vi "PhotonPoseEstimator_Execute.vi"(7 "Configuration":T12={"Primary Strategy"=enum."LOWEST_AMBIGUITY", "Camera"="", "Initial Pose"={"Translation3d"={"X"=0.0, "Y"=0.0, "Z"=0.0}, "Rotation3d"={"Q_quaternion"={"R"=1.0, "V"=[0.0, 0.0, 0.0]}}}, "HighestAmbiguity"=0.0, "RobotToCamera"={"TRANSLATION3D"={"X"=0.0, "Y"=0.0, "Z"=0.0}, "ROTATION3D"={"Q_quaternion"={"R"=1.0, "V"=[0.0, 0.0, 0.0]}}, "XF"=FALSE}, "FallBack Strategy"=enum."LOWEST_AMBIGUITY", "BaseNTName"="/photonvision"} {"RobotToCamera"."TRANSLATION3D"."Z" format="%14.3f"; "RobotToCamera"."TRANSLATION3D"."Y" format="%14.3f"; "RobotToCamera"."TRANSLATION3D"."X" format="%14.3f"; "Initial Pose"."Translation3d"."Z" format="%14.3f"; "Initial Pose"."Translation3d"."Y" format="%14.3f"; "Initial Pose"."Translation3d"."X" format="%14.3f"}, 8 "AprilTagFieldLayout":T1={"AprilTagMap"={}, "FieldLength"=0.0, "FieldWidth"=0.0, "OriginPosition "=enum."kBlueAllianceWallRightSide,", "OriginPose3d"={"Translation3d"={"X"=0.0, "Y"=0.0, "Z"=0.0}, "Rotation3d"={"Q_quaternion"={"R"=1.0, "V"=[0.0, 0.0, 0.0]}}}} {"OriginPose3d"."Translation3d"."Z" format="%14.3f"; "OriginPose3d"."Translation3d"."Y" format="%14.3f"; "OriginPose3d"."Translation3d"."X" format="%14.3f"}, 9 "ReferencePose":T3={"Translation3d"={"X"=0.0, "Y"=0.0, "Z"=0.0}, "Rotation3d"={"Q_quaternion"={"R"=1.0, "V"=[0.0, 0.0, 0.0]}}} {"Translation3d"."Z" format="%14.3f"; "Translation3d"."Y" format="%14.3f"; "Translation3d"."X" format="%14.3f"}, 10 "PIpeline Has \nNew Results":bool, 11 "PipelineResult":T14={"Targets"=[], "PhotonMultiTargetPNPResult"={"PhotonPNPResult"={"IsPresent"=FALSE, "bestReprojErr"=0.0, "altReprojErr"=0.0, "ambiguity"=0.0, "Best"={"TRANSLATION3D"={"X"=0.0, "Y"=0.0, "Z"=0.0}, "ROTATION3D"={"Q_quaternion"={"R"=1.0, "V"=[0.0, 0.0, 0.0]}}, "XF"=FALSE}, "Alt"={"TRANSLATION3D"={"X"=0.0, "Y"=0.0, "Z"=0.0}, "ROTATION3D"={"Q_quaternion"={"R"=1.0, "V"=[0.0, 0.0, 0.0]}}, "XF"=FALSE}}, "FiducialIDsUsed"=[]}, "PhotonPipelineMetadata"={"CaptureTimestampMicros"=0, "PublishTimestampMicros"=0, "SequenceID"=0, "TimeSinceLastPong"=0}} {"PhotonMultiTargetPNPResult"."PhotonPNPResult"."Alt"."TRANSLATION3D"."Z" format="%14.3f"; "PhotonMultiTargetPNPResult"."PhotonPNPResult"."Alt"."TRANSLATION3D"."Y" format="%14.3f"; "PhotonMultiTargetPNPResult"."PhotonPNPResult"."Alt"."TRANSLATION3D"."X" format="%14.3f"; "PhotonMultiTargetPNPResult"."PhotonPNPResult"."Best"."TRANSLATION3D"."Z" format="%14.3f"; "PhotonMultiTargetPNPResult"."PhotonPNPResult"."Best"."TRANSLATION3D"."Y" format="%14.3f"; "PhotonMultiTargetPNPResult"."PhotonPNPResult"."Best"."TRANSLATION3D"."X" format="%14.3f"; "Targets"."AltCameraToTarget"."TRANSLATION3D"."Z" format="%14.3f"; "Targets"."AltCameraToTarget"."TRANSLATION3D"."Y" format="%14.3f"; "Targets"."AltCameraToTarget"."TRANSLATION3D"."X" format="%14.3f"; "Targets"."BestCameraToTarget"."TRANSLATION3D"."Z" format="%14.3f"; "Targets"."BestCameraToTarget"."TRANSLATION3D"."Y" format="%14.3f"; "Targets"."BestCameraToTarget"."TRANSLATION3D"."X" format="%14.3f"}) -> (0 "TimeStamp_Seconds":dbl, 1 "New Pose Found":bool, 2 "EstimatedPose2d":T8={"TRANSLATION"={"X"=0.0, "Y"=0.0}, "ROTATION"={"VALUE"=0.0, "COS"=1.0, "SIN"=0.0}} {"ROTATION"."SIN" format="%13.4f"; "ROTATION"."COS" format="%13.4f"; "ROTATION"."VALUE" format="%13.4f"; "TRANSLATION"."Y" format="%14.3f"; "TRANSLATION"."X" format="%14.3f"}, 3 "EstimatedPose3d":T3={"Translation3d"={"X"=0.0, "Y"=0.0, "Z"=0.0}, "Rotation3d"={"Q_quaternion"={"R"=1.0, "V"=[0.0, 0.0, 0.0]}}} {"Translation3d"."Z" format="%14.3f"; "Translation3d"."Y" format="%14.3f"; "Translation3d"."X" format="%14.3f"}, 4 "Strategy Used":T11, 5 "PhotonEstimatedRobotPose":T20={"EstimatedPose"={"Translation3d"={"X"=0.0, "Y"=0.0, "Z"=0.0}, "Rotation3d"={"Q_quaternion"={"R"=1.0, "V"=[0.0, 0.0, 0.0]}}}, "TimeStamp_Seconds"=0.0, "targetsUsed"=[], "Strategy"=enum."LOWEST_AMBIGUITY"} {"targetsUsed"."AltCameraToTarget"."TRANSLATION3D"."Z" format="%14.3f"; "targetsUsed"."AltCameraToTarget"."TRANSLATION3D"."Y" format="%14.3f"; "targetsUsed"."AltCameraToTarget"."TRANSLATION3D"."X" format="%14.3f"; "targetsUsed"."BestCameraToTarget"."TRANSLATION3D"."Z" format="%14.3f"; "targetsUsed"."BestCameraToTarget"."TRANSLATION3D"."Y" format="%14.3f"; "targetsUsed"."BestCameraToTarget"."TRANSLATION3D"."X" format="%14.3f"; "EstimatedPose"."Translation3d"."Z" format="%14.3f"; "EstimatedPose"."Translation3d"."Y" format="%14.3f"; "EstimatedPose"."Translation3d"."X" format="%14.3f"}, 6 "out PhotonPoseEstimator":T21={"LastPose"={"Translation3d"={"X"=0.0, "Y"=0.0, "Z"=0.0}, "Rotation3d"={"Q_quaternion"={"R"=1.0, "V"=[0.0, 0.0, 0.0]}}}, "ReferencePose"={"Translation3d"={"X"=0.0, "Y"=0.0, "Z"=0.0}, "Rotation3d"={"Q_quaternion"={"R"=1.0, "V"=[0.0, 0.0, 0.0]}}}, "FieldTags"={"AprilTagMap"={}, "FieldLength"=0.0, "FieldWidth"=0.0, "OriginPosition "=enum."kBlueAllianceWallRightSide,", "OriginPose3d"={"Translation3d"={"X"=0.0, "Y"=0.0, "Z"=0.0}, "Rotation3d"={"Q_quaternion"={"R"=1.0, "V"=[0.0, 0.0, 0.0]}}}}, "PrimaryStratety"=enum."LOWEST_AMBIGUITY", "Camera"="", "RobotToCamera"={"TRANSLATION3D"={"X"=0.0, "Y"=0.0, "Z"=0.0}, "ROTATION3D"={"Q_quaternion"={"R"=1.0, "V"=[0.0, 0.0, 0.0]}}, "XF"=FALSE}, "ReportedErrors"=[], "HighestAmbiguity"=10.0, "MultiTagFallbackStrategy"=enum."LOWEST_AMBIGUITY", "PoseCacheTimeoutSec"=-1.0, "PhotonTargetModel"={"Vertices"=[], "IsPlaner"=FALSE, "IsSpherical"=FALSE}, "BaseNTName"="/photonvision", "HeadingBuffer"={"TimeStamps"=[], "RotationValues"=[], "Min_TimeStamp"=0.0, "Max_TimeStamp"=0.0, "ItemCount"=0, "MaxBufferTime"=0.0}} {"HeadingBuffer"."RotationValues"."SIN" format="%13.4f"; "HeadingBuffer"."RotationValues"."COS" format="%13.4f"; "HeadingBuffer"."RotationValues"."VALUE" format="%13.4f"; "PhotonTargetModel"."Vertices"."Z" format="%14.3f"; "PhotonTargetModel"."Vertices"."Y" format="%14.3f"; "PhotonTargetModel"."Vertices"."X" format="%14.3f"; "RobotToCamera"."TRANSLATION3D"."Z" format="%14.3f"; "RobotToCamera"."TRANSLATION3D"."Y" format="%14.3f"; "RobotToCamera"."TRANSLATION3D"."X" format="%14.3f"; "FieldTags"."OriginPose3d"."Translation3d"."Z" format="%14.3f"; "FieldTags"."OriginPose3d"."Translation3d"."Y" format="%14.3f"; "FieldTags"."OriginPose3d"."Translation3d"."X" format="%14.3f"; "ReferencePose"."Translation3d"."Z" format="%14.3f"; "ReferencePose"."Translation3d"."Y" format="%14.3f"; "ReferencePose"."Translation3d"."X" format="%14.3f"; "LastPose"."Translation3d"."Z" format="%14.3f"; "LastPose"."Translation3d"."Y" format="%14.3f"; "LastPose"."Translation3d"."X" format="%14.3f"})   [LabVIEW 2019, in "PhotonVisionLib.lvlib"]
doc: "Provided data from polling a camera, update the estimated position of the robot. Returns empty if there are no cameras set or no targets were found from the cameras. \n\nInputs:\n -- PhotonPoseEstimator -- data cluster -- Data guiding how the position determination is done.\n -- PipelineResults -- data cluster -- Data provided from PhotonCamera_GetLatestResults.\n -- HasResults -- boolean - TRUE if targets have been identified in the Pipeline results. This can be provided by PhotonCamera_GetLatestResults.\n -- AprilTagFieldLayout -- data cluster -- Field layout defining the location of April Tags\n\nOutputs:\n - EstimatedPose3d - Pose3d - Estimated 3d position. Only value if NewPoseFound = TRUE\n - EstimatedPose2d - Pose2d - Estimated 2d position. Only value if NewPoseFound = TRUE\n - NewPoseFound -- boolean -- A new position has been determined.\n - TimeStampe - double - Target timestamp (seconds)\n - StrategyUsed -- enum -- The strategy used to determine the pose.\n - PhotonEstimatedRobotPose -- data cluster -- Complete estimated robot position and timestamp data cluster\n -- PhotonPoseEstimator -- data cluster -- Updated data cluster."
uses:
  PhotonVisionLib.lvlib
  TypeDef/PhotonPoseEstimatorType.ctl
  <vilib>/Rock Robotics/WPI/ThirdParty/JAS_Junk/TrajLib/TypeDef/POSE3D.ctl
  <vilib>/Rock Robotics/WPI/ThirdParty/JAS_Junk/TrajLib/TypeDef/TRANSLATION3D.ctl
  <vilib>/Rock Robotics/WPI/ThirdParty/JAS_Junk/TrajLib/TypeDef/ROTATION3D.ctl
  <vilib>/Rock Robotics/WPI/ThirdParty/JAS_Junk/TrajLib/TypeDef/QUATERNION.ctl
  <vilib>/Rock Robotics/WPI/ThirdParty/JAS_Junk/TrajLib/TypeDef/AprilTagFieldLayout.ctl
  <vilib>/Rock Robotics/WPI/ThirdParty/JAS_Junk/TrajLib/TypeDef/AprilTag.ctl
  <vilib>/Rock Robotics/WPI/ThirdParty/JAS_Junk/TrajLib/Enum/AprilTagFieldLayoutOrignPosition_ENUM.ctl
  Enum/PhotonPoseStrategy_ENUM.ctl
  <vilib>/Rock Robotics/WPI/ThirdParty/JAS_Junk/TrajLib/TypeDef/TRANSFORM3D.ctl
  TypeDef/PhotonTargetModel.ctl
  <vilib>/Rock Robotics/WPI/ThirdParty/JAS_Junk/TrajLib/TypeDef/TIME_INTERPOLATABLE_ROTATION2D.ctl
  <vilib>/Rock Robotics/WPI/ThirdParty/JAS_Junk/TrajLib/TypeDef/ROTATION2D.ctl
  TypeDef/PhotonEstimatedRobotPoseType.ctl
  TypeDef/PhotonTrackedTargetType.ctl
  TypeDef/TargetCornerType.ctl
  TypeDef/PhotonPipelineResultType.ctl
  TypeDef/PhotonMultiTargetPNPResultType.ctl
  TypeDef/PhotonPNPResultType.ctl
  TypeDef/PhotonPipelineMetadataType.ctl
  TypeDef/PhotonPoseEstimator_Configuration.ctl
  <vilib>/Rock Robotics/WPI/ThirdParty/JAS_Junk/TrajLib/TypeDef/POSE2D.ctl
  <vilib>/Rock Robotics/WPI/ThirdParty/JAS_Junk/TrajLib/TypeDef/TRANSLATION2D.ctl
  <vilib>/Rock Robotics/WPI/ThirdParty/JAS_Junk/TrajLib/VI/Transform3d_GetTranslation3d.vi
  <vilib>/Rock Robotics/WPI/ThirdParty/JAS_Junk/TrajLib/VI/Transform3d_GetRotation3d.vi
  <vilib>/Rock Robotics/WPI/ThirdParty/JAS_Junk/TrajLib/VI/Rotation3d_Equals.vi
  <vilib>/Rock Robotics/WPI/ThirdParty/JAS_Junk/TrajLib/VI/Translation3d_Equals.vi
  PhotonTargetModel_New_AprilTag36H11.vi
  <vilib>/Rock Robotics/WPI/ThirdParty/JAS_Junk/TrajLib/VI/TimeInterpRotation2d_New.vi
  PhotonPoseEstimator_Update_All.vi
  <vilib>/Rock Robotics/WPI/ThirdParty/JAS_Junk/TrajLib/VI/Pose3d_getTranslation3d.vi
  <vilib>/Rock Robotics/WPI/ThirdParty/JAS_Junk/TrajLib/VI/Pose3d_getRotation3d.vi
  <vilib>/Rock Robotics/WPI/ThirdParty/JAS_Junk/TrajLib/VI/Translation3d_ToTranslation2d.vi
  <vilib>/Rock Robotics/WPI/ThirdParty/JAS_Junk/TrajLib/VI/Rotation3d_ToRotation2d.vi
  <vilib>/Rock Robotics/WPI/ThirdParty/JAS_Junk/TrajLib/Pose2d_New_TRRO.vi
  <vilib>/Rock Robotics/WPI/ThirdParty/JAS_Junk/TrajLib/VI/Rotation3d_GetQuaterion.vi
  <vilib>/Rock Robotics/WPI/ThirdParty/JAS_Junk/TrajLib/VI/Quaternion_Equals.vi
  PhotonTargetModel_New_RectPlanar.vi
  <vilib>/Rock Robotics/WPI/ThirdParty/JAS_Junk/TrajLib/Conv_Inches_Meters.vi
  PhotonPoseEstimator_GetEmptyPose.vi
  PhotonPoseEstimator_Strategy_lowestAmbiguity.vi
  PhotonPoseEstimator_Strategy_closestToCameraHeight.vi
  PhotonPoseEstimator_Strategy_closestToReferencePose.vi
  PhotonPoseEstimator_GetReferencePose.vi
  PhotonPoseEstimator_GetLastPose.vi
  PhotonPoseEstimator_Strategy_averageBestTargets.vi
  PhotonPoseEstimator_Strategy_multiTagOnCoproc.vi
  PhotonPoseEstimator_Strategy_pnpDistanceTrigSolve.vi
  PhotonPoseEstimator_Strategy_constrainedPnpStrategy.vi
  PhotonPipelineResult_GetTimeStampSecs.vi
  <vilib>/Rock Robotics/WPI/ThirdParty/JAS_Junk/TrajLib/Translation2d_Create.vi
  <vilib>/Rock Robotics/WPI/ThirdParty/JAS_Junk/TrajLib/Rotation2d_CreateAngle.vi
  <vilib>/Rock Robotics/WPI/ThirdParty/JAS_Junk/TrajLib/VI/Rotation3d_GetXYZ.vi
  <vilib>/Rock Robotics/WPI/ThirdParty/JAS_Junk/TrajLib/VI/Quaternion_Get_Vect.vi
  <vilib>/Rock Robotics/WPI/ThirdParty/JAS_Junk/TrajLib/VI/Quaternion_Get_W.vi
  <vilib>/Rock Robotics/WPI/ThirdParty/JAS_Junk/TrajLib/VI/Translation3d_Create.vi
  PhotonTargetModel_New.vi
  <vilib>/Rock Robotics/WPI/ThirdParty/JAS_Junk/TrajLib/VI/Rotation3d_Create_AxisAngle.vi
  <vilib>/Rock Robotics/WPI/ThirdParty/JAS_Junk/TrajLib/VI/Pose3d_New.vi
  PhotonPipelineResult_HasTargets.vi
  PhotonPipelineResult_GetTargets.vi
  PhotonTrackedTarget_GetPoseAmbiguity.vi
  PhotonTrackedTarget_GetFiducialId.vi
  PhotonPoseEstimator_GetFieldTags.vi
  <vilib>/Rock Robotics/WPI/ThirdParty/JAS_Junk/TrajLib/VI/AprilTagFieldLayout_GetTagPose.vi
  <vilib>/Rock Robotics/WPI/ThirdParty/JAS_Junk/TrajLib/VI/Pose3d_TransformBy.vi
  PhotonTrackedTarget_GetBestCameraToTarget.vi
  <vilib>/Rock Robotics/WPI/ThirdParty/JAS_Junk/TrajLib/VI/Transform3d_Inverse.vi
  PhotonPoseEstimator_GetRobotToCameraTransform.vi
  PhotonPoseEstimator_GetHighestAmbiguity.vi
  PhotonEstimatedRobotPose_New.vi
  PhotonPoseEstimator_Strategy_closestToCameraHeight_calc.vi
  PhotonTrackedTarget_GetAltCameraToTarget.vi
  PhotonPoseEstimator_Strategy_closestToReferencePose_calc.vi
  PhotonPoseEstimator_Strategy_averageBestTargets_calc.vi
  <vilib>/Rock Robotics/WPI/ThirdParty/JAS_Junk/TrajLib/VI/Rotation3d_Plus.vi
  <vilib>/Rock Robotics/WPI/ThirdParty/JAS_Junk/TrajLib/VI/Translation3d_Plus.vi
  <vilib>/Rock Robotics/WPI/ThirdParty/JAS_Junk/TrajLib/VI/Translation3d_Times.vi
  <vilib>/Rock Robotics/WPI/ThirdParty/JAS_Junk/TrajLib/VI/Rotation3d_Times.vi
  <vilib>/Rock Robotics/WPI/ThirdParty/JAS_Junk/TrajLib/VI/Rotation3d_Create_Default.vi
  <vilib>/Rock Robotics/WPI/ThirdParty/JAS_Junk/TrajLib/VI/Translation3d_Create_Default.vi
  <vilib>/Rock Robotics/WPI/ThirdParty/JAS_Junk/TrajLib/VI/Pose3d_New_Trans3dRot3d.vi
  <vilib>/Rock Robotics/WPI/ThirdParty/JAS_Junk/TrajLib/VI/Pose3d_New_Default.vi
  <vilib>/Rock Robotics/WPI/ThirdParty/JAS_Junk/TrajLib/VI/Pose3d_Plus.vi
  <vilib>/Rock Robotics/WPI/ThirdParty/JAS_Junk/TrajLib/VI/Pose3d_RelativeTo.vi
  <vilib>/Rock Robotics/WPI/ThirdParty/JAS_Junk/TrajLib/VI/AprilTagFieldLayout_GetOriginPosition.vi
  PhotonPipelineResult_GetMultiTagResult.vi
  <vilib>/Rock Robotics/WPI/ThirdParty/JAS_Junk/TrajLib/VI/Quaternion_Get_All.vi
  <vilib>/Rock Robotics/WPI/ThirdParty/JAS_Junk/TrajLib/VI/Quaternion_New.vi
  <vilib>/Rock Robotics/WPI/ThirdParty/JAS_Junk/TrajLib/VI/Vector_Norm.vi
  <vilib>/Rock Robotics/WPI/ThirdParty/JAS_Junk/TrajLib/VecBuilder_ArrayBy1Fill.vi
  <vilib>/Rock Robotics/WPI/ThirdParty/JAS_Junk/TrajLib/VI/AprilTag_GetAll.vi
  <vilib>/Rock Robotics/WPI/ThirdParty/JAS_Junk/TrajLib/VI/Translation3d_RotateBy.vi
  <vilib>/Rock Robotics/WPI/ThirdParty/JAS_Junk/TrajLib/Transform2d_Create_TransRot.vi
  <vilib>/Rock Robotics/WPI/ThirdParty/JAS_Junk/TrajLib/VI/Transform3d_Create_Trans3dRot3d.vi
  <vilib>/Rock Robotics/WPI/ThirdParty/JAS_Junk/TrajLib/VI/Rotation3d_UnaryMinus.vi
  <vilib>/Rock Robotics/WPI/ThirdParty/JAS_Junk/TrajLib/VI/Translation3d_UnaryMinus.vi
  <vilib>/Rock Robotics/WPI/ThirdParty/JAS_Junk/TrajLib/VI/Transform3d_GetXYZ.vi
  <vilib>/Rock Robotics/WPI/ThirdParty/JAS_Junk/TrajLib/VI/Pose3d_getXYZ.vi
  PhotonPoseEstimator_CalcDifference.vi
  <vilib>/Rock Robotics/WPI/ThirdParty/JAS_Junk/TrajLib/VI/Rotation3d_RotateBy.vi
  <vilib>/Rock Robotics/WPI/ThirdParty/JAS_Junk/TrajLib/VI/Translation3d_GetXYZ.vi
  <vilib>/Rock Robotics/WPI/ThirdParty/JAS_Junk/TrajLib/VI/Quaternion_New_Default.vi
  <vilib>/Rock Robotics/WPI/ThirdParty/JAS_Junk/TrajLib/VI/Transform3d_Create_Pose3dPose3d.vi
  <vilib>/Rock Robotics/WPI/ThirdParty/JAS_Junk/TrajLib/MatBuilder_Create.vi
  <vilib>/Rock Robotics/WPI/ThirdParty/JAS_Junk/TrajLib/VI/Quaternion_Times.vi
  <vilib>/Rock Robotics/WPI/ThirdParty/JAS_Junk/TrajLib/VI/Quaternion_Inverse.vi
  <vilib>/Rock Robotics/WPI/ThirdParty/JAS_Junk/TrajLib/VI/Rotation3d_Create_Quaternion.vi
  <vilib>/Rock Robotics/WPI/ThirdParty/JAS_Junk/TrajLib/VI/Translation3d_GetDistance.vi
  <vilib>/Rock Robotics/WPI/ThirdParty/JAS_Junk/TrajLib/VI/Translation3d_Minus.vi
  <vilib>/Rock Robotics/WPI/ThirdParty/JAS_Junk/TrajLib/VI/Rotation3d_Minus.vi
  <vilib>/Rock Robotics/WPI/ThirdParty/JAS_Junk/TrajLib/VI/Quaternion_Normalize.vi
  <vilib>/Rock Robotics/WPI/ThirdParty/JAS_Junk/TrajLib/Trajectory_Library.lvlib
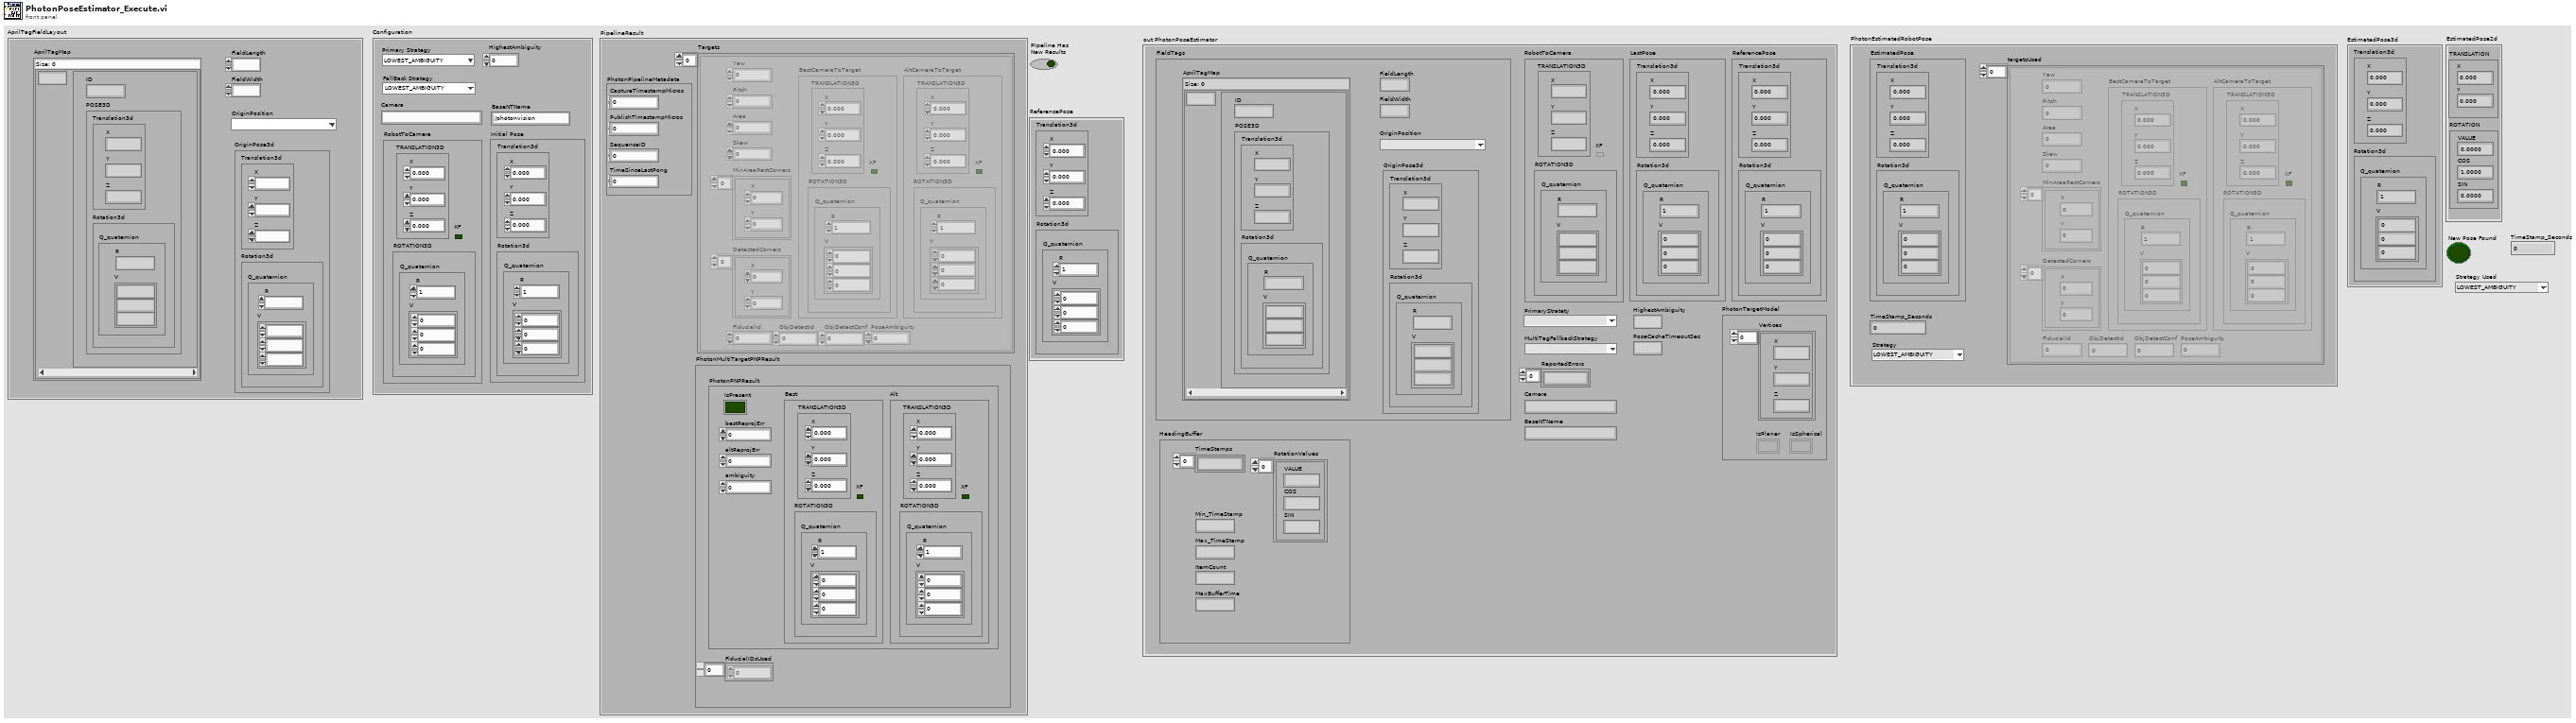
[diagram p1: front panel]
types:
  T1 = typedef "Trajectory_Library.lvlib/AprilTagFieldLayout.ctl" = cluster{"AprilTagMap":map{i32, T2}, "FieldLength":dbl, "FieldWidth":dbl, "OriginPosition ":T7, "OriginPose3d":T3}
  T2 = typedef "Trajectory_Library.lvlib/AprilTag.ctl" = cluster{"ID":i32, "POSE3D":T3}
  T3 = typedef "Trajectory_Library.lvlib/POSE3D.ctl" = cluster{"Translation3d":T4, "Rotation3d":T5}
  T4 = typedef "Trajectory_Library.lvlib/TRANSLATION3D.ctl" = cluster{"X":dbl, "Y":dbl, "Z":dbl}
  T5 = typedef "Trajectory_Library.lvlib/ROTATION3D.ctl" = cluster{"Q_quaternion":T6}
  T6 = typedef "Trajectory_Library.lvlib/QUATERNION.ctl" = cluster{"R":dbl, "V":dbl[]}
  T7 = typedef "Trajectory_Library.lvlib/AprilTagFieldLayoutOrignPosition_ENUM.ctl" = enum16{"kBlueAllianceWallRightSide,", "kRedAllianceWallRightSide,"}
  T8 = typedef "Trajectory_Library.lvlib/POSE2D.ctl" = cluster{"TRANSLATION":T9, "ROTATION":T10}
  T9 = typedef "Trajectory_Library.lvlib/TRANSLATION2D.ctl" = cluster{"X":dbl, "Y":dbl}
  T10 = typedef "Trajectory_Library.lvlib/ROTATION2D.ctl" = cluster{"VALUE":dbl, "COS":dbl, "SIN":dbl}
  T11 = typedef "PhotonVisionLib.lvlib/PhotonPoseStrategy_ENUM.ctl" = enum16{"LOWEST_AMBIGUITY", "CLOSEST_TO_CAMERA_HEIGHT", "CLOSEST_TO_REFERENCE_POSE", "CLOSEST_TO_LAST_POSE", "AVERAGE_BEST_TARGETS", "MULTI_TAG_PNP_ON_COPROCESSOR", "MULTI_TAG_PNP_ON_RIO", "PNP_DISTANCE_TRIG_SOLVE", "CONSTRAINED_SOLVEPNP"}
  T12 = typedef "PhotonVisionLib.lvlib/PhotonPoseEstimator_Configuration.ctl" = cluster{"Primary Strategy":T11, "Camera":string, "Initial Pose":T3, "HighestAmbiguity":dbl, "RobotToCamera":T13, "FallBack Strategy":T11, "BaseNTName":string}
  T13 = typedef "Trajectory_Library.lvlib/TRANSFORM3D.ctl" = cluster{"TRANSLATION3D":T4, "ROTATION3D":T5, "XF":bool}
  T14 = typedef "PhotonVisionLib.lvlib/PhotonPipelineResultType.ctl" = cluster{"Targets":T15[], "PhotonMultiTargetPNPResult":T17, "PhotonPipelineMetadata":T19}
  T15 = typedef "PhotonVisionLib.lvlib/PhotonTrackedTargetType.ctl" = cluster{"Yaw":dbl, "Pitch":dbl, "Area":dbl, "Skew":dbl, "MinAreaRectCorners":T16[], "BestCameraToTarget":T13, "FiducialId":i32, "AltCameraToTarget":T13, "PoseAmbiguity":dbl, "DetectedCorners":T16[], "ObjDetectId":i32, "ObjDetectConf":sgl}
  T16 = typedef "PhotonVisionLib.lvlib/TargetCornerType.ctl" = cluster{"X":dbl, "Y":dbl}
  T17 = typedef "PhotonVisionLib.lvlib/PhotonMultiTargetPNPResultType.ctl" = cluster{"PhotonPNPResult":T18, "FiducialIDsUsed":i16[]}
  T18 = typedef "PhotonVisionLib.lvlib/PhotonPNPResultType.ctl" = cluster{"IsPresent":bool, "bestReprojErr":dbl, "altReprojErr":dbl, "ambiguity":dbl, "Best":T13, "Alt":T13}
  T19 = typedef "PhotonVisionLib.lvlib/PhotonPipelineMetadataType.ctl" = cluster{"CaptureTimestampMicros":i64, "PublishTimestampMicros":i64, "SequenceID":i64, "TimeSinceLastPong":i64}
  T20 = typedef "PhotonVisionLib.lvlib/PhotonEstimatedRobotPoseType.ctl" = cluster{"EstimatedPose":T3, "TimeStamp_Seconds":dbl, "targetsUsed":T15[], "Strategy":T11}
  T21 = typedef "PhotonVisionLib.lvlib/PhotonPoseEstimatorType.ctl" = cluster{"LastPose":T3, "ReferencePose":T3, "FieldTags":T1, "PrimaryStratety":T11, "Camera":string, "RobotToCamera":T13, "ReportedErrors":dbl[], "HighestAmbiguity":dbl, "MultiTagFallbackStrategy":T11, "PoseCacheTimeoutSec":dbl, "PhotonTargetModel":T22, "BaseNTName":string, "HeadingBuffer":T23}
  T22 = typedef "PhotonVisionLib.lvlib/PhotonTargetModel.ctl" = cluster{"Vertices":T4[], "IsPlaner":bool, "IsSpherical":bool}
  T23 = typedef "Trajectory_Library.lvlib/TIME_INTERPOLATABLE_ROTATION2D.ctl" = cluster{"TimeStamps":dbl[], "RotationValues":T10[], "Min_TimeStamp":dbl, "Max_TimeStamp":dbl, "ItemCount":i32, "MaxBufferTime":dbl}
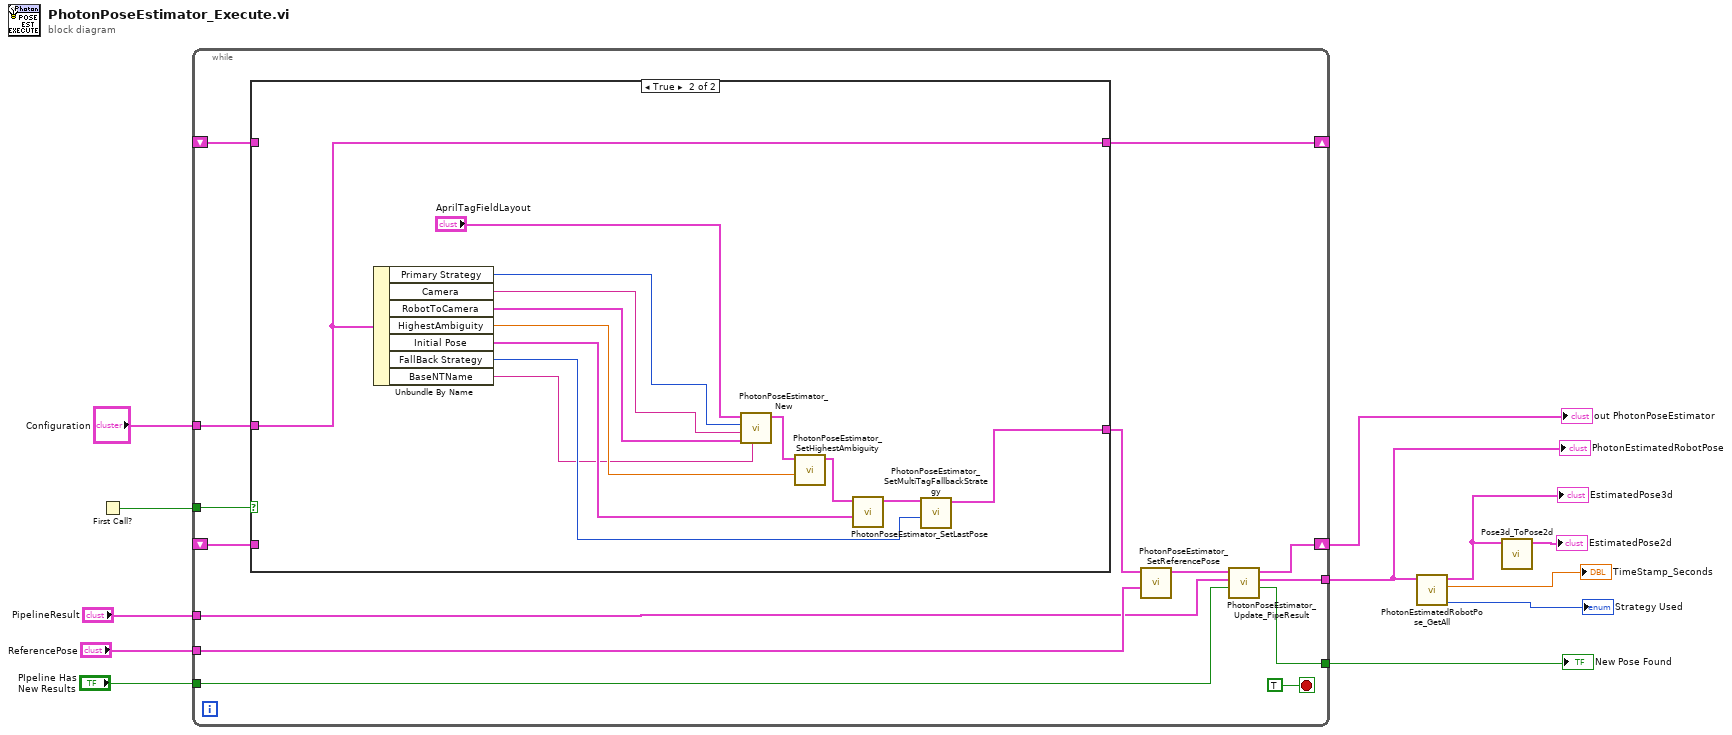
[diagram p0: block diagram]
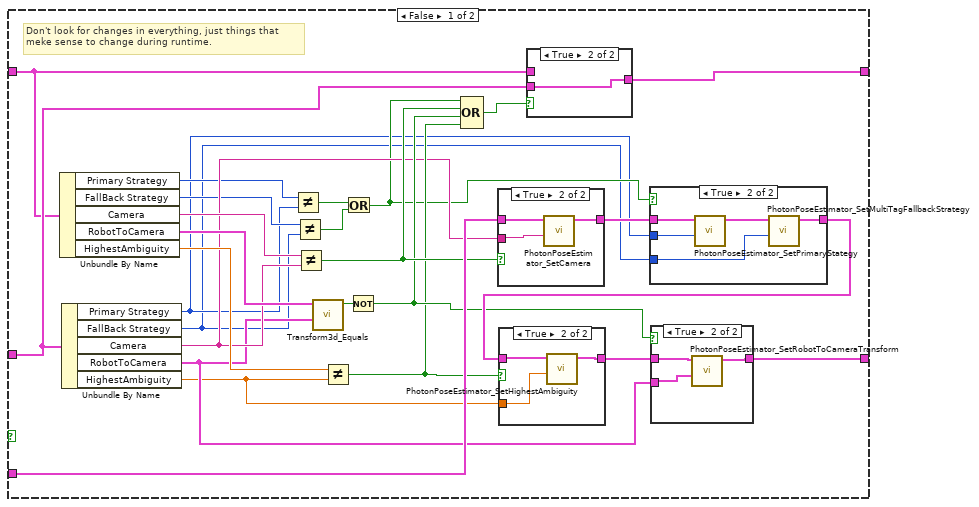
[diagram p2: hidden frame]
diagram:
  n1 = First Call?() -> (First Call?: T/F=w12:bool)
  n2 = while {
    tunnel: w12 -> [w13]
    tunnel: "PipelineResult" -> [w22]
    shift-right: [w20] -> w8
    shift-left: _ -> [w25]
    tunnel: "ReferencePose" -> [w24]
    tunnel: "PIpeline Has \nNew Results" -> [w21]
    tunnel: [w19] -> w5
    tunnel: [w17] -> w7
    tunnel: "Configuration" -> [w15]
    shift-right: [w16] -> _
    shift-left: _ -> [w14]
    stop <- TRUE stop-if-true
    n3 = case shown="True" w13 {
      tunnel: [w34 w76] -> w18
      tunnel: w25 -> [w46 _]
      tunnel: w15 -> [w49 w78]
      tunnel: [w47 w78] -> w16
      tunnel: w14 -> [w48 _]
      frame False {
        # "Don't look for changes in everything, just things that\nmeke sense to change during runtime."
        n4 = Unbundle By Name(w48) -> ("Primary Strategy"=w30:T11, "FallBack Strategy"=w29:T11, "Camera"=w43:string, "RobotToCamera"=w39:T13, "HighestAmbiguity"=w52:dbl)
        n5 = Unbundle By Name(w49) -> ("Primary Strategy"=w28:T11, "FallBack Strategy"=w27:T11, "Camera"=w37:string, "RobotToCamera"=w36:T13, "HighestAmbiguity"=w35:dbl)
        n6 = Not Equal?(x=w30, y=w28) -> (x != y?=w32:bool)
        n7 = Not Equal?(x=w29, y=w27) -> (x != y?=w31:bool)
        n8 = Not Equal?(x=w43, y=w37) -> (x != y?=w44:bool)
        n9 = call <vilib>:"Transform3d_Equals.vi"("otherTransform3d"=w36, "inTransform3d"=w39) -> ("Equals"=w51:bool)  [unwired: 9 in]
        n10 = Not Equal?(x=w52, y=w35) -> (x != y?=w38:bool)
        n11 = Or(x=w32, y=w31) -> (x .or. y?=w33:bool)
        n12 = Not(x=w51) -> (.not. x?=w40:bool)
        n13 = Compound Arithmetic op=OR(w33, w44, w40, w38) -> (w50:bool)
        n14 = case shown="True" w44 {
          tunnel: w46 -> [w69 w72]
          tunnel: [w69 w71] -> w45
          tunnel: w37 -> [_ w70]
          frame False {
          }
          frame True {
            n15 = call "PhotonPoseEstimator_SetCamera.vi"("Camera"=w70, "PhotonPoseEstimator"=w72) -> ("out PhotonPoseEstimator"=w71:T21)  [unwired: 9 in]
          }
        }
        n16 = case shown="True" w50 {
          tunnel: w49 -> [_ w68]
          tunnel: w48 -> [w67 _]
          tunnel: [w67 w68] -> w47
          frame False {
          }
          frame True {
          }
        }
        n17 = case shown="True" w33 {
          tunnel: w45 -> [w61 w66]
          tunnel: w28 -> [_ w65]
          tunnel: [w61 w63] -> w41
          tunnel: w27 -> [_ w62]
          frame False {
          }
          frame True {
            n18 = call "PhotonPoseEstimator_SetPrimaryStategy.vi"("PrimaryStrategy"=w65, "PhotonPoseEstimator"=w66) -> ("out PhotonPoseEstimator"=w64:T21)  [unwired: 9 in]
            n19 = call "PhotonPoseEstimator_SetMultiTagFallbackStrategy.vi"("FallBack Strategy"=w62, "PhotonPoseEstimator"=w64) -> ("out PhotonPoseEstimator"=w63:T21)  [unwired: 9 in]
          }
        }
        n20 = case shown="True" w38 {
          tunnel: w41 -> [w57 w60]
          tunnel: [w57 w59] -> w42
          tunnel: w35 -> [_ w58]
          frame False {
          }
          frame True {
            n21 = call "PhotonPoseEstimator_SetHighestAmbiguity.vi"("HighestAmbiguity"=w58, "PhotonPoseEstimator"=w60) -> ("out PhotonPoseEstimator"=w59:T21)  [unwired: 9 in]
          }
        }
        n22 = case shown="True" w40 {
          tunnel: w42 -> [w53 w56]
          tunnel: [w53 w55] -> w34
          tunnel: w36 -> [_ w54]
          frame False {
          }
          frame True {
            n23 = call "PhotonPoseEstimator_SetRobotToCameraTransform.vi"("RobotToCameraTransform3d"=w54, "PhotonPoseEstimator"=w56) -> ("out PhotonPoseEstimator"=w55:T21)  [unwired: 9 in]
          }
        }
      }
      frame True {
        n24 = Unbundle By Name(w78) -> ("Primary Strategy"=w83:T11, "Camera"=w82:string, "RobotToCamera"=w81:T13, "HighestAmbiguity"=w80:dbl, "Initial Pose"=w79:T3, "FallBack Strategy"=w75:T11, "BaseNTName"=w74:string)
        n25 = call "PhotonPoseEstimator_New.vi"("BaseNTName"=w74, "RobotToCamera"=w81, "Camera"=w82, "Strategy"=w83, "AprilTagFieldLayout"="AprilTagFieldLayout") -> ("PhotonPoseEstimator"=w85:T21)  [unwired: 6 in]
        n26 = call "PhotonPoseEstimator_SetHighestAmbiguity.vi"("HighestAmbiguity"=w80, "PhotonPoseEstimator"=w85) -> ("out PhotonPoseEstimator"=w84:T21)  [unwired: 9 in]
        n27 = call "PhotonPoseEstimator_SetLastPose.vi"("LastPose"=w79, "PhotonPoseEstimator"=w84) -> ("out PhotonPoseEstimator"=w77:T21)  [unwired: 9 in]
        n28 = call "PhotonPoseEstimator_SetMultiTagFallbackStrategy.vi"("FallBack Strategy"=w75, "PhotonPoseEstimator"=w77) -> ("out PhotonPoseEstimator"=w76:T21)  [unwired: 9 in]
      }
    }
    n29 = call "PhotonPoseEstimator_SetReferencePose.vi"("ReferencePose"=w24, "PhotonPoseEstimator"=w18) -> ("out PhotonPoseEstimator"=w23:T21)  [unwired: 9 in]
    n30 = call "PhotonPoseEstimator_Update_PipeResult.vi"("Has Results"=w21, "PipelineResult"=w22, "PhotonPoseEstimator"=w23) -> ("Pos Found"=w17:bool, "PhotonEstimatedRobotPose"=w19:T20, "out PhotonPoseEstimator"=w20:T21)  [unwired: 6 in]
  }
  "out PhotonPoseEstimator" <- w8
  "PhotonEstimatedRobotPose" <- w5
  "New Pose Found" <- w7
  n31 = call "PhotonEstimatedRobotPose_GetAll.vi"("PhotonEstimatedRobotPose"=w5) -> ("Strategy"=→"Strategy Used":T11, "TimeStamp_Seconds"=→"TimeStamp_Seconds":dbl, "EstimatedPose"=w3:T3)  [unwired: 7 in, 1 out]
  "EstimatedPose3d" <- w3
  n32 = call <vilib>:"Pose3d_ToPose2d.vi"("in Pose3d"=w3) -> ("out Pose2d"=→"EstimatedPose2d":T8)  [unwired: 10 in]
